vi "PH_Periodic_Sequencer.PC StateSeqSM.vi"(0 "i ref in":refnum<vi>, 2 "SM State":string, 3 "not linked?":bool, 5 "error in (no error)":errorcluster) -> (14 "i ref out":refnum<vi>, 19 "error out":errorcluster)   [LabVIEW 2014, in "PH_Periodic_Sequencer.lvlib"]
doc: "This VI writes the Sequencer SM state to the GUI and own attributes."
uses:
  PH_Periodic_Sequencer.lvlib
  PH_Basics/PH_Common/PH_Common.lvlib
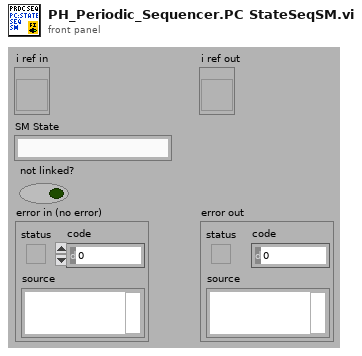
[diagram p1: front panel]
types:
  T1 = typedef "PH_Periodic_Sequencer.lvlib/PH_Periodic_Sequencer.i attribute.ctl" = cluster{"GUI Refs":cluster{"Main Off":refnum<vi>, "Start":refnum<vi>, "Ready":refnum<vi>, "Sequencer SM State":refnum<vi>, "Interval [sec]":refnum<vi>, "Wanted Shots":refnum<vi>, "Delivered Shots":refnum<vi>}, "PU Info":cluster{"Instancename":string, "State":T2, "linked":bool}[], "Sequencer":cluster{"Instancename":string, "linked?":bool, "R2S?":bool, "SM State":string}, "Run?":bool, "Interval [sec]":dbl, "PU State Refs":refnum<vi>[], "Wanted Shots":i32, "Delivered Shots":i32}
  T2 = typedef "PH_StatusHandler.lvlib/PH_StatusHandler.Status.ctl" = i16
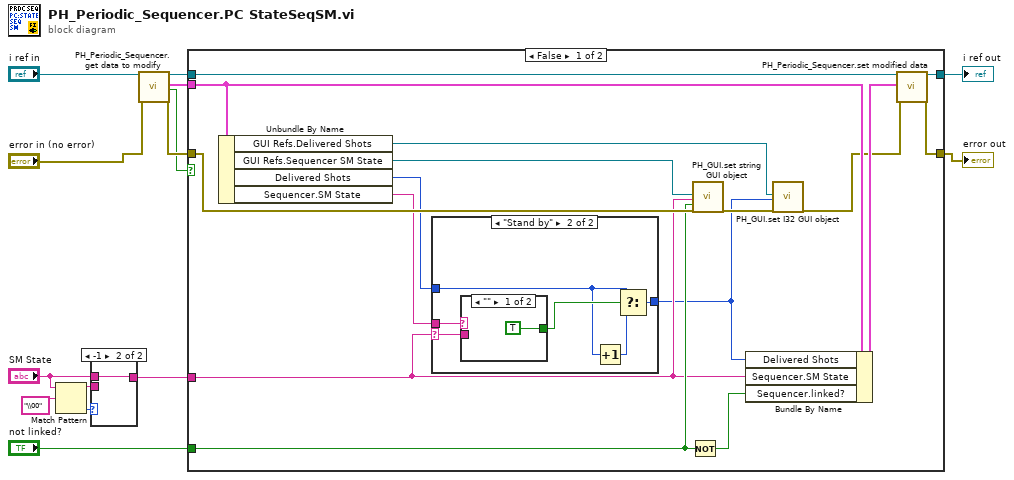
[diagram p0: block diagram]
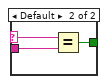
[diagram p3: hidden frame]
diagram:
  n1 = Match Pattern(string="SM State", regular expression="\\00" ("search string")) -> (before substring=w5:string, offset past match=w6:i32)  [unwired: 1 in, 2 out]
  n2 = case shown="-1" w6 {
    tunnel: [w15 w16] -> w2
    tunnel: "SM State" -> [_ w16]
    tunnel: w5 -> [w15 _]
    frame Default {
    }
    frame -1 {
    }
  }
  n3 = call "PH_Periodic_Sequencer.get data to modify.vi"("i ref in"="i ref in", "error in (no error)"="error in (no error)") -> ("i ref out"=w9:refnum<vi>, "i attribute"=w14:T1, "timed out"=w3:bool, "error out"=w11:errorcluster)  [unwired: 14 in]
  n4 = case shown="False" w3 {
    tunnel: w14 -> [w27 _]
    tunnel: w11 -> [w31 w44]
    tunnel: [w30 w44] -> w10
    tunnel: w9 -> [w29 w45]
    tunnel: [w28 w45] -> w8
    tunnel: w2 -> [w23 _]
    tunnel: "not linked?" -> [w25 _]
    frame False {
      n5 = Unbundle By Name(w27) -> ("GUI Refs.Delivered Shots"=w18:refnum<vi>, "GUI Refs.Sequencer SM State"=w32:refnum<vi>, "Delivered Shots"=w22:i32, "Sequencer.SM State"=w21:string)
      n6 = case shown="\"Stand by\"" w23 {
        selector: w23 -> [_ w39]
        tunnel: w22 -> [w33 w36]
        tunnel: w21 -> [_ w34]
        tunnel: [w33 w37] -> w17
        frame Default {
        }
        frame "Stand by" {
          n7 = case shown="\"\"" w34 {
            selector: w34 -> [_ w41]
            tunnel: w39 -> [_ w43]
            tunnel: [TRUE w42] -> w38
            frame "" {
            }
            frame Default {
              n8 = Equal?(x=w41, y=w43) -> (x = y?=w42:bool)
            }
          }
          n9 = Increment(x=w36) -> (x+1=w35:i32)
          n10 = Select(t=w36, s=w38, f=w35) -> (s? t:f=w37:i32)
        }
      }
      n11 = Not(x=w25) -> (.not. x?=w24:bool)
      n12 = call "PH_GUI.set string GUI object.vi"("GUI object Ref"=w32, "Text"=w23, "Blinking? (false)"=w25, "error in"=w31) -> ("error out"=w20:errorcluster)  [unwired: 15 in]
      n13 = Bundle By Name(cluster=w27, "Delivered Shots"=w17, "Sequencer.SM State"=w23, "Sequencer.linked?"=w24) -> (w26:T1)
      n14 = call "PH_GUI.set I32 GUI object.vi"("I32 GUI Ref"=w18, "value"=w17, "error in (no error)"=w20) -> ("error out"=w19:errorcluster)  [unwired: 16 in]
      n15 = call "PH_Periodic_Sequencer.set modified data.vi"("i ref in"=w29, "i attribute"=w26, "error in (no error)"=w19) -> ("i ref out"=w28:refnum<vi>, "error out"=w30:errorcluster)  [unwired: 15 in]
    }
    frame True {
    }
  }
  "error out" <- w10
  "i ref out" <- w8
